vi "User Events - Init.vi"(8 "error in (no error)":errorcluster) -> (0 "error out":errorcluster, 3 "UE Data Container":T1)   [LabVIEW 2017]
doc: "Initialize all user events for ATM Controller."
uses:
  UE Data Container.ctl
  Error Handler/Controls/Error Data.ctl
  UIs/User Console/Controls/User Console - Transaction Enum.ctl
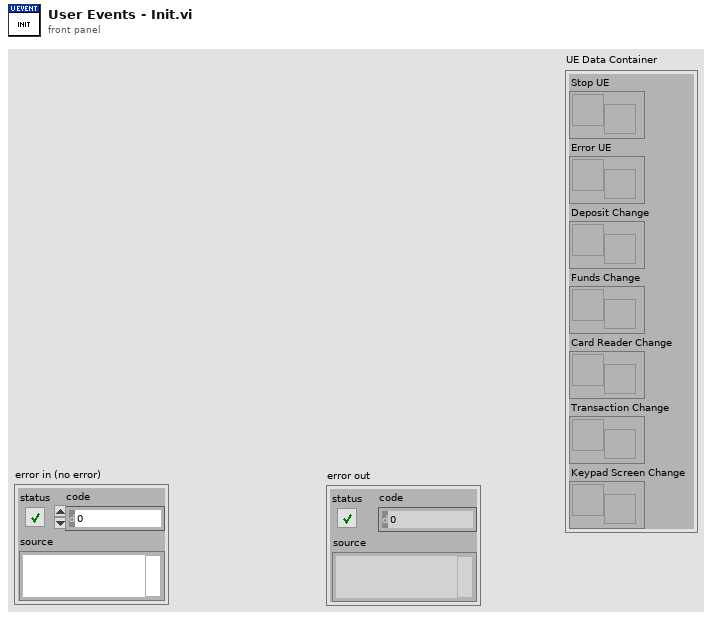
[diagram p1: front panel]
types:
  T1 = typedef "UE Data Container.ctl" = cluster{"Stop UE":refnum<user-event>, "Error UE":refnum<user-event>, "Deposit Change":refnum<user-event>, "Funds Change":refnum<user-event>, "Card Reader Change":refnum<user-event>, "Transaction Change":refnum<user-event>, "Keypad Screen Change":refnum<user-event>}
  T2 = typedef "User Console - Transaction Enum.ctl" = enum16{"Balance Inquiry", "Deposit", "Withdrawal", "Fat Cash", "New Transaction", "Terminate Session"}
  T3 = typedef "Error Data.ctl" = cluster{"Type":enum16{"Console Error", "Sensor Interface IO Error", "Process Step Error"}, "Data":variant}
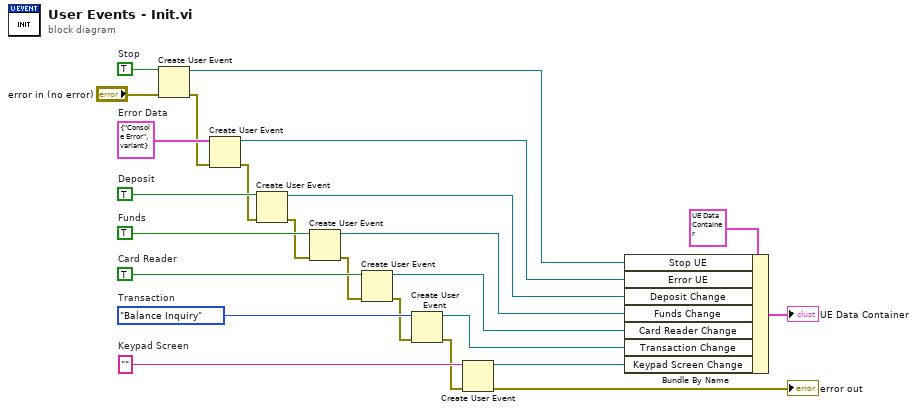
[diagram p0: block diagram]
diagram:
  w11 = ""  # Keypad Screen
  w13 = User_Console_-_Transaction_Enum."Balance Inquiry"  # Transaction
  w15 = TRUE  # Card Reader
  w17 = TRUE  # Funds
  w19 = TRUE  # Deposit
  w21 = T3 {"Type"=enum."Console Error", "Data"=variant}  # Error Data
  w23 = TRUE  # Stop
  n1 = Create User Event(user event datatype=w23, error in="error in (no error)") -> (user event=w2:refnum<user-event>, error out=w20:errorcluster)
  n2 = Create User Event(user event datatype=w21, error in=w20) -> (user event=w3:refnum<user-event>, error out=w18:errorcluster)
  n3 = Create User Event(user event datatype=w19, error in=w18) -> (user event=w4:refnum<user-event>, error out=w16:errorcluster)
  n4 = Create User Event(user event datatype=w17, error in=w16) -> (user event=w5:refnum<user-event>, error out=w14:errorcluster)
  n5 = Create User Event(user event datatype=w15, error in=w14) -> (user event=w6:refnum<user-event>, error out=w12:errorcluster)
  n6 = Create User Event(user event datatype=w13, error in=w12) -> (user event=w7:refnum<user-event>, error out=w10:errorcluster)
  n7 = Create User Event(user event datatype=w11, error in=w10) -> (user event=w9:refnum<user-event>, error out=→"error out":errorcluster)
  n8 = Bundle By Name(cluster=T1 {"Stop UE"=refnum, "Error UE"=refnum, "Deposit Change"=refnum, "Funds Change"=refnum, "Card Reader Change"=refnum, "Transaction Change"=refnum, "Keypad Screen Change"=refnum} ("UE Data Container"), "Stop UE"=w2, "Error UE"=w3, "Deposit Change"=w4, "Funds Change"=w5, "Card Reader Change"=w6, "Transaction Change"=w7, "Keypad Screen Change"=w9) -> (→"UE Data Container":T1)
